vi "try_TDMS File Viewer.vi"() -> ()   [LabVIEW 2020]
uses:
  <vilib>/Utility/TDMS File Viewer/NI_TDMS File Viewer.lvlib
panel:
  in  "Stop":bool
  in  "Button":bool
  in  "Sample files":i32(listbox)
  # "Scenario\nThe TDMS File Viewer has a refreshed appearance and improved performance. This tool is useful for browsing the data stored in a TDMS file. You can drop the TDMS File Viewer with Quick Drop.\n\nInstructions\n1. Run the VI\n2. Select the TDMS file you want to display from the preloaded Sample Files \n3. Click on Launch TDMS Viewer Button"
  # "Close this VI when you are done with the demo."
  # "You do not need to save changes to this VI."
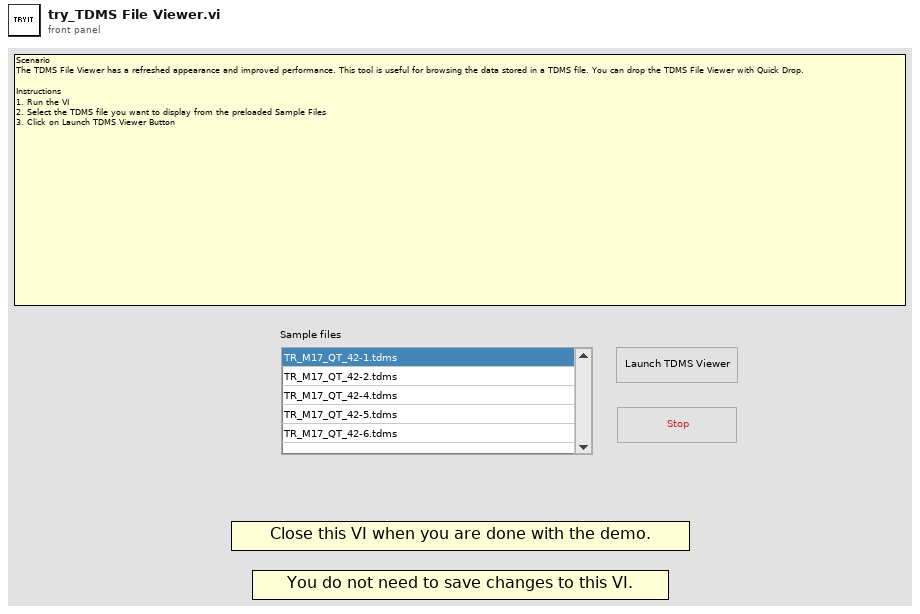
[diagram p1: front panel]
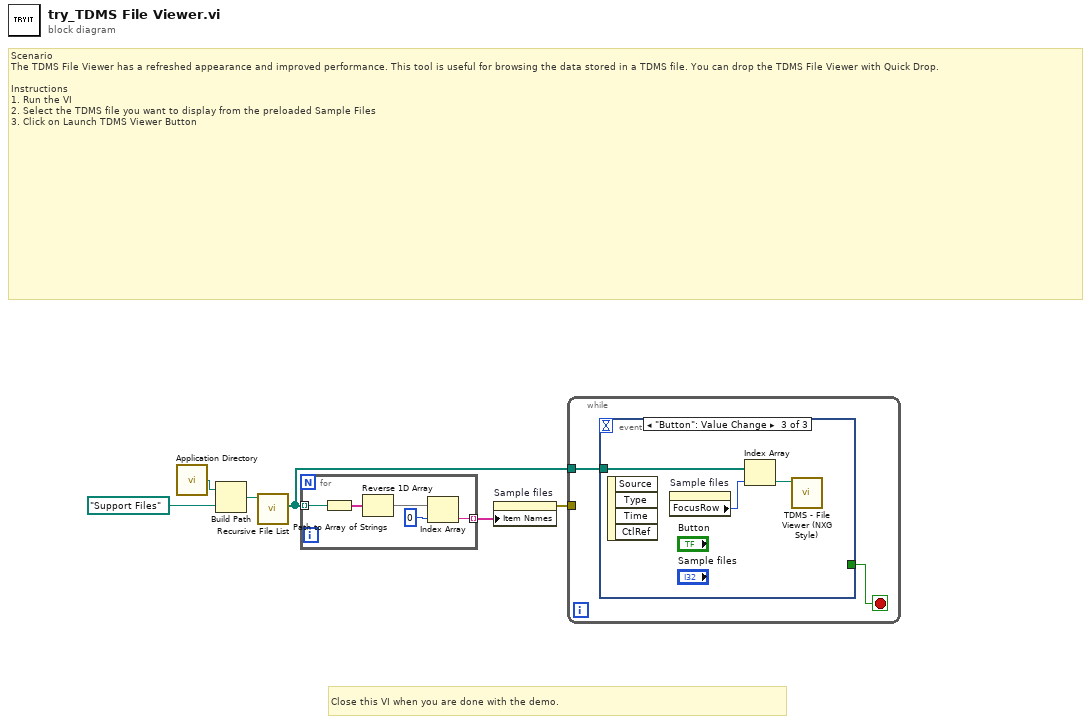
[diagram p0: block diagram]
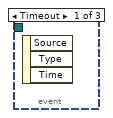
[diagram p2: hidden frame]
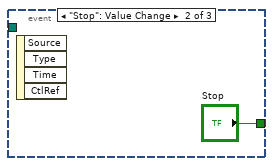
[diagram p3: hidden frame]
diagram:
  # "Close this VI when you are done with the demo."
  # "Scenario\nThe TDMS File Viewer has a refreshed appearance and improved performance. This tool is useful for browsing the data stored in a TDMS file. You can drop the TDMS File Viewer with Quick Drop.\n\nInstructions\n1. Run the VI\n2. Select the TDMS file you want to display from the preloaded Sample Files \n3. Click on Launch TDMS Viewer Button"
  n1 = call <vilib>:"Application Directory.vi"() -> ("Application Directory"=w6:path)
  n2 = Build Path(base path=w6, name or relative path=path "Support Files") -> (appended path=w4:path)
  n3 = call <vilib>:"Recursive File List.vi"("Folder Path"=w4) -> ("All Files in Dir"=w2:path[])  [unwired: 6 in, 4 out]
  n4 = for {
    tunnel: w2 -> [w11] mode=indexing
    tunnel: [w7] -> w3 mode=indexing
    n5 = Path to Array of Strings(0:w11) -> (2:w10:string[])  [unwired: 1 out]
    n6 = Reverse 1D Array(array=w10) -> (reversed array=w9:string[])
    n7 = Index Array(array=w9, index=0) -> (element=w7:string)
  }
  n8 = property on="Sample files" class="LstBox (strict)"("Item Names"=w3) -> (error out=w1:errorcluster)  [unwired: 2 in, 1 out]
  n9 = while {
    tunnel: w2 -> [w12]
    tunnel: w1 -> [_]
    stop <- w13 stop-if-true
    n10 = event shown="[2] \"Button\": Value Change" {
      selector: _ -> [_ _ _]
      dyn-events: _ -> [_ _ _]
      timeout: _ -> [_ _ _]
      tunnel: [_ "Stop" _] -> w13
      tunnel: w12 -> [_ _ w17]
      event Timeout {
        n11 = event-data() -> ()  [unwired: 1 in, 3 out]
      }
      event "Stop": Value Change {
        n12 = event-data() -> ()  [unwired: 1 in, 4 out]
      }
      event "Button": Value Change {
        n13 = event-data() -> ()  [unwired: 1 in, 4 out]
        n14 = property on="Sample files" class="LstBox (strict)"() -> ("FocusRow"=w16:i32)  [unwired: 2 in, 2 out]
        n15 = Index Array(array=w17, index=w16) -> (element=w15:path)
        n16 = call <vilib>:"TDMS - File Viewer (NXG Style).vi"("file in"=w15) -> ()  [unwired: 9 in, 2 out]
      }
    }
  }
